vi "ActOnResult.vi"(0 "ActionLvDialog in":refnum<class "ActionLvDialog.lvclass">, 1 "Data":variant, 5 "error in (no error)":errorcluster) -> (14 "ActionLvDialog out":refnum<class "ActionLvDialog.lvclass">, 19 "error out":errorcluster)   [LabVIEW 2017, in "ActionLvDialog.lvclass"]
doc: "Base class implementation (empty)."
uses:
  ActionLvDialog.lvclass
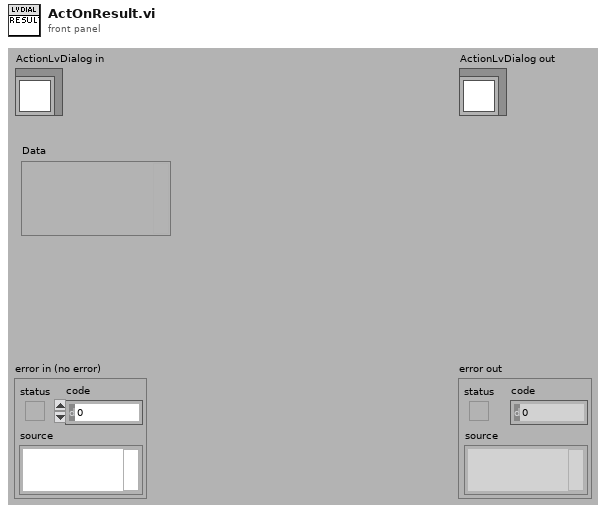
[diagram p1: front panel]
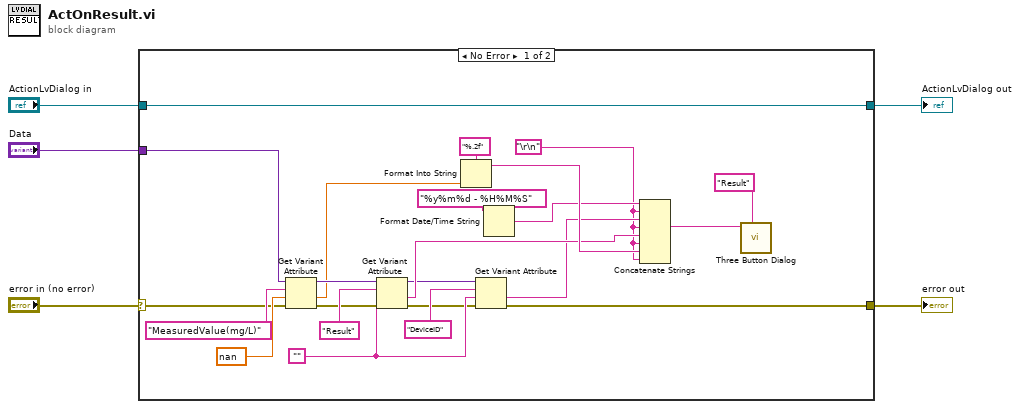
[diagram p0: block diagram]
diagram:
  n1 = case shown="No Error" "error in (no error)" {
    selector: "error in (no error)" -> [w13 w29]
    tunnel: "ActionLvDialog in" -> [w14 w30]
    tunnel: [w14 w30] -> w4
    tunnel: [w12 w29] -> w2
    tunnel: "Data" -> [w11 _]
    frame No Error {
      w6 = "\r\n" ("format string")
      w20 = ""
      n2 = Get Variant Attribute(Variant=w11, name="MeasuredValue(mg/L)", default value (empty Variant)=nan, error in=w13) -> (duplicate Variant=w23:variant, value=w18:dbl, error out=w21:errorcluster)  [unwired: 1 out]
      n3 = Get Variant Attribute(Variant=w23, name="Result", default value (empty Variant)=w20, error in=w21) -> (duplicate Variant=w9:variant, value=w17:string, error out=w10:errorcluster)  [unwired: 1 out]
      n4 = Format Into String(format string="%.2f", w18) -> (resulting string=w26:string)  [unwired: 2 in, 1 out]
      n5 = Get Variant Attribute(Variant=w9, name="DeviceID", default value (empty Variant)=w20, error in=w10) -> (value=w15:string, error out=w12:errorcluster)  [unwired: 2 out]
      n6 = Format Date/Time String(time format string (%c)="%y%m%d - %H%M%S") -> (date/time string=w16:string)  [unwired: 1 in, 1 out]
      n7 = Concatenate Strings(w16, w6, w15, w6, w17, w6, w26, w6) -> (w8:string)
      n8 = call <vilib>:"Three Button Dialog.vi"("Window Title (\"\")"="Result" ("Window Title (\"\")"), "message"=w8) -> ()  [unwired: 9 in, 1 out]
    }
    frame Error {
    }
  }
  "error out" <- w2
  "ActionLvDialog out" <- w4
